vi "ProgramControlLogEvent.vi"(0 "Universal Robot.lvclass":refnum<class "Universal Robot.lvclass">, 5 "data":variant, 8 "Event Type":T1, 9 "Program":string) -> (14 "Universal Robot.lvclass out":refnum<class "Universal Robot.lvclass">)   [LabVIEW 2019, in "Universal Robot.lvclass"]
uses:
  Universal Robot.lvclass
  Events/Robot Event/Event Type.ctl
  Universal Robot.lvclass/Universal Robot.ctl
  Events/Robot Event/Robot Event.lvclass
panel:
  out "Errors (unhandled)":errorcluster[](array[cluster])
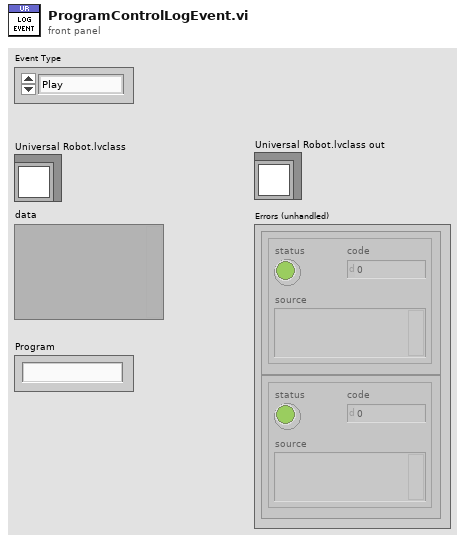
[diagram p1: front panel]
types:
  T1 = typedef "Robot Event.lvclass/Event Type.ctl" = enum16{"Play", "Error", "Fault", "Timeout", "Stopped", "Complete", "Fault - Program Resumed", "Fault - Program Aborted"}
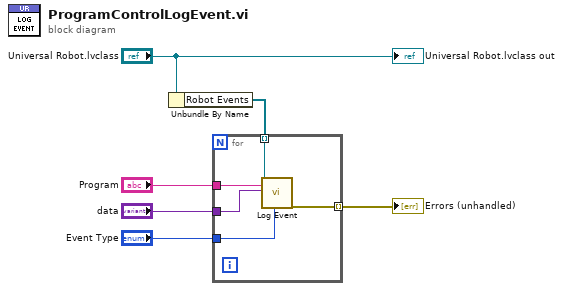
[diagram p0: block diagram]
diagram:
  n1 = Unbundle By Name("Universal Robot.lvclass") -> ("Robot Events"=w5:refnum<class "Robot Event.lvclass">[])
  n2 = for {
    tunnel: w5 -> [w11] mode=indexing
    tunnel: "Program" -> [w10]
    tunnel: "data" -> [w9]
    tunnel: "Event Type" -> [w8]
    tunnel: [w7] -> w1 mode=indexing
    n3 = call-dynamic "Log Event.vi"("Robot Notifications in"=w11, "Program"=w10, "data"=w9, "Event Type"=w8) -> ("error out"=w7:errorcluster)  [unwired: 14 in, 1 out]
  }
  "Errors (unhandled)" <- w1
  "Universal Robot.lvclass out" <- "Universal Robot.lvclass"
